vi "tb_02-periode.vi"(0 "Etude":T2, 1 "Booléen":bool, 5 "VS":T4, 7 "ent-2D":string[][](array[string]), 9 "do-2D":string[][](array[string]), 11 "tb in ?":bool[](array[boolean])) -> (4 "Etude":T2, 6 "VS":T4, 8 "ent-2D":T1[][](array[typedef]), 10 "do-2D":string[][](array[string]), 12 "Per":string[](array[string]), 13 "Pér-ent":T1, 14 "Pér-lib":T1, 15 "tb in ?":bool[](array[boolean]))   [LabVIEW 2010, in "lv_04.lvlib"]
uses:
  lv_04/lv_04.lvlib
  lv_04/commandes/cX.ctl
  lv_04/commandes/cSTA_varid.ctl
  lv_04/commandes/c_TDMS_ch_variable.ctl
  lv_04/commandes/c_TDMS_ch_donnees.ctl
  lv_04/commandes/c0-var-n.ctl
  lv_04/commandes/cSTA_num_do_cr.ctl
  lv_04/commandes/c02-do-num.ctl
  lv_04/commandes/c04-stat-num.ctl
  lv_04/commandes/cSTA_txt_do_cr.ctl
  lv_04/commandes/c02-do-txt.ctl
  lv_04/commandes/c04-stat-txt.ctl
  lv_04/commandes/cSTA_dist.ctl
  lv_04/commandes/c03-dist-S.ctl
  lv_04/commandes/c0-dist-xy.ctl
  lv_04/commandes/c03-dist-T.ctl
  lv_04/commandes/c03-dist-SPC.ctl
  lv_04/commandes/c_etude.ctl
  lv_02/p_5E_ch_loi.ctl
  lv_01/lv_01.lvlib
  lv_02/lv_02.lvlib
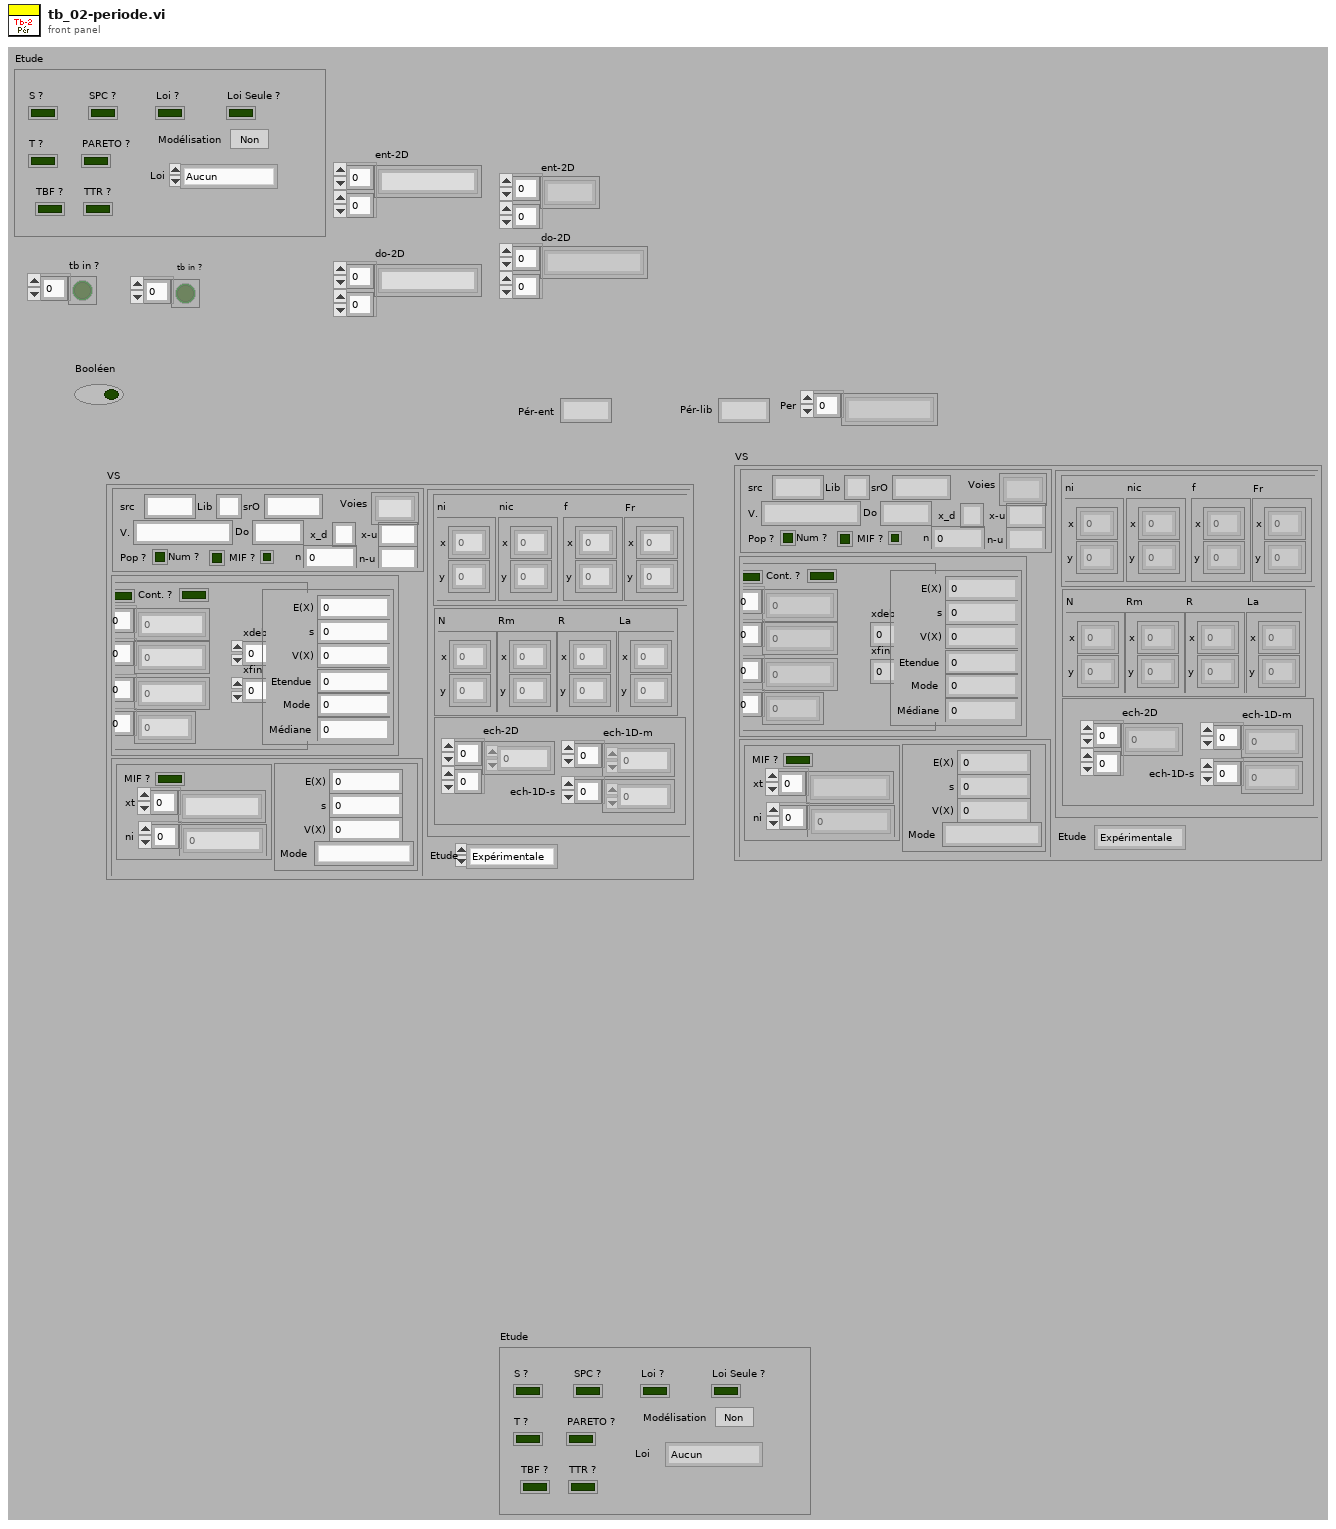
[diagram p1: front panel]
types:
  T1 = typedef "lv_04.lvlib/c_TDMS_ch_donnees.ctl" = string
  T2 = typedef "lv_04.lvlib/c_etude.ctl" = cluster{"T ?":bool, "S ?":bool, "SPC ?":bool, "PARETO ?":bool, "TBF ?":bool, "TTR ?":bool, "Loi ?":bool, "Loi Seule ?":bool, "Modélisation":bool, "Loi":T3}
  T3 = typedef "lv_02.lvlib/p_5E_ch_loi.ctl" = enum16{"Aucun", "Normale", "Aucun2", "Aucun3", "Binômial", "Poisson", "Exponentiel", "Weibull", "Rang médian"}
  T4 = typedef "lv_04.lvlib/cX.ctl" = cluster{"src":T5, "num":T8, "txt":T11, "dist":T14, "Etude":enum16{"Expérimentale", "Modèle"}}
  T5 = typedef "lv_04.lvlib/cSTA_varid.ctl" = cluster{"src":string, "Lib":string, "srO":string, "V.":T6, "Voies":string[], "Do":T1, "n":T7, "Num ?":bool, "Pop ?":bool, "x_d":string, "x-u":string, "n-u":string, "MIF ?":bool}
  T6 = typedef "lv_04.lvlib/c_TDMS_ch_variable.ctl" = string
  T7 = typedef "lv_04.lvlib/c0-var-n.ctl" = i32
  T8 = typedef "lv_04.lvlib/cSTA_num_do_cr.ctl" = cluster{"do":T9, "sta":T10}
  T9 = typedef "lv_04.lvlib/c02-do-num.ctl" = cluster{"MIF ?":bool, "Cont. ?":bool, "xi":dbl[], "xic":dbl[], "ni":u32[], "dx":dbl[], "xdeb":dbl, "xfin":dbl}
  T10 = typedef "lv_04.lvlib/c04-stat-num.ctl" = cluster{"E(X)":dbl, "s":dbl, "V(X) ":dbl, "Etendue":dbl, "Mode":dbl, "Médiane":dbl}
  T11 = typedef "lv_04.lvlib/cSTA_txt_do_cr.ctl" = cluster{"do":T12, "sta":T13}
  T12 = typedef "lv_04.lvlib/c02-do-txt.ctl" = cluster{"xt":string[], "ni":dbl[], "MIF ?":bool}
  T13 = typedef "lv_04.lvlib/c04-stat-txt.ctl" = cluster{"E(X)":dbl, "s":dbl, "V(X) ":dbl, "Mode":string}
  T14 = typedef "lv_04.lvlib/cSTA_dist.ctl" = cluster{"S":T15, "T":T17, "spc":T18}
  T15 = typedef "lv_04.lvlib/c03-dist-S.ctl" = cluster{"nic":T16, "f":T16, "Fr":T16, "ni":T16}
  T16 = typedef "lv_04.lvlib/c0-dist-xy.ctl" = cluster{"x":dbl[], "y":dbl[]}
  T17 = typedef "lv_04.lvlib/c03-dist-T.ctl" = cluster{"N":T16, "Rm":T16, "R":T16, "La":T16}
  T18 = typedef "lv_04.lvlib/c03-dist-SPC.ctl" = cluster{"ech-2D":dbl[][], "ech-1D-m":dbl[], "ech-1D-s":dbl[]}
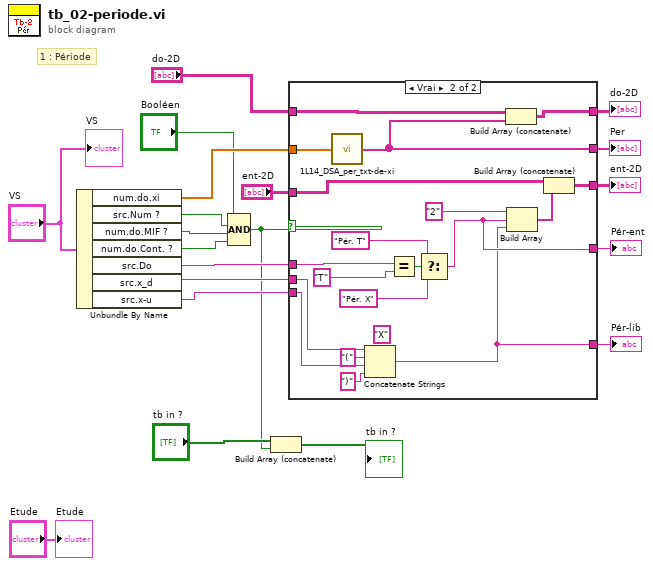
[diagram p0: block diagram]
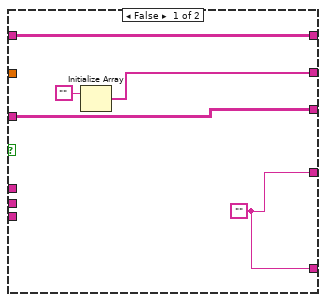
[diagram p2: hidden frame]
diagram:
  # "1 : Période"
  n1 = Unbundle By Name("VS") -> ("num.do.xi"=w15:dbl[], "src.Num ?"=w18:bool, "num.do.MIF ?"=w17:bool, "num.do.Cont. ?"=w16:bool, "src.Do"=w11:T1, "src.x_d"=w12:string, "src.x-u"=w13:string)
  n2 = Compound Arithmetic op=AND("Booléen", w18, w17, w16) -> (w1:bool)
  n3 = Build Array (concatenate)("tb in ?", w1) -> (→"tb in ?":bool[])
  n4 = case shown="Vrai" w1 {
    tunnel: w15 -> [_ w44]
    tunnel: [w25 w42] -> w14
    tunnel: w13 -> [_ w28]
    tunnel: w12 -> [_ w31]
    tunnel: w11 -> [_ w32]
    tunnel: "do-2D" -> [w23 w43]
    tunnel: [w23 w41] -> w9
    tunnel: "ent-2D" -> [w22 w40]
    tunnel: [w22 w38] -> w7
    tunnel: [w21 w27] -> w6
    tunnel: [w21 w26] -> w5
    frame False {
      w21 = ""
      n5 = Initialize Array("") -> (w25:string[])  [unwired: 1 in]
    }
    frame True {
      (unwired) T1 "X" ("y")
      n6 = call "1L14_DSA_per_txt-de-xi.vi"("xi"=w44) -> ("Période"=w42:string[])
      n7 = Concatenate Strings(w31, "(" ("chaîne"), w28, ")" ("chaîne")) -> (w26:string)
      n8 = Equal?(x=w32, y=T1 "T") -> (x = y?=w33:bool)
      n9 = Select(t="Pér. T", s=w33, f="Pér. X") -> (s? t:f=w27:string)
      n10 = Build Array (concatenate)(w43, w42) -> (w41:string[][])
      n11 = Build Array("2", w27, w26) -> (w39:string[])
      n12 = Build Array (concatenate)(w40, w39) -> (w38:string[][])
    }
  }
  "Per" <- w14
  "Pér-ent" <- w6
  "Pér-lib" <- w5
  "ent-2D" <- w7
  "do-2D" <- w9
  "VS" <- "VS"
  "Etude" <- "Etude"
